vi "Init.vi"(8 "error in (no error)":errorcluster caption="错误输入（无错误）", 10 "Url":string, 11 "HttpClient 输入":refnum<class "HttpClient.lvclass"> caption="DNL_LabVIEW Object in") -> (0 "error out":errorcluster caption="错误输出", 3 "HttpClient 输出":refnum<class "HttpClient.lvclass"> caption="DNL_LabVIEW Object out")   [LabVIEW 2012, in "HttpClient.lvclass"]
uses:
  HttpClient.lvclass
  HttpClient.lvclass/HttpClient.ctl
  Libs/Http/Http.lvclass
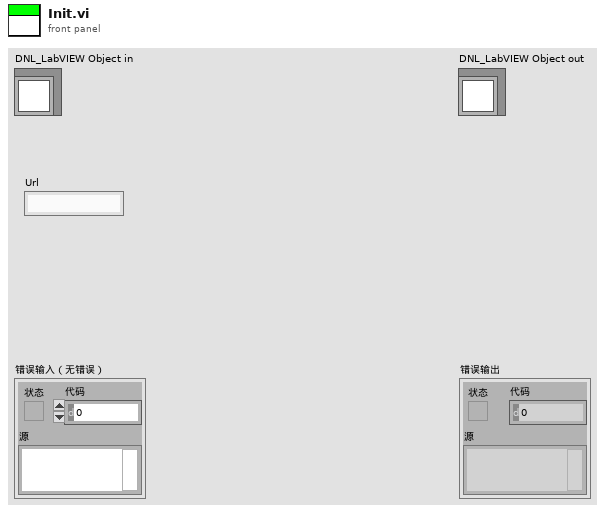
[diagram p1: front panel]
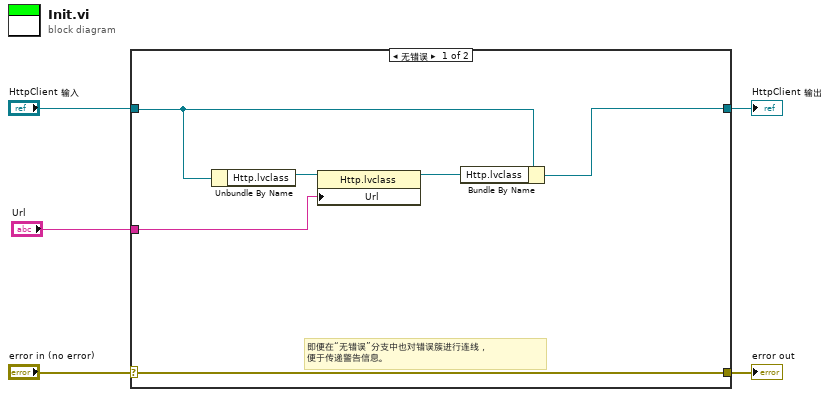
[diagram p0: block diagram]
diagram:
  n1 = case shown="无错误" "error in (no error)" {
    selector: "error in (no error)" -> [w11 w13]
    tunnel: [w11 w13] -> w4
    tunnel: [w6 w12] -> w2
    tunnel: "HttpClient 输入" -> [w10 w12]
    tunnel: "Url" -> [w7 _]
    frame No Error {
      # "即便在“无错误”分支中也对错误簇进行连线，\n便于传递警告信息。"
      n2 = Unbundle By Name(w10) -> ("Http.lvclass"=w9:refnum<class "Http.lvclass">)
      n3 = property class="Http.lvclass"(reference=w9, "Url"=w7) -> (reference out=w8:refnum<class "Http.lvclass">)  [unwired: 1 in, 1 out]
      n4 = Bundle By Name(cluster=w10, "Http.lvclass"=w8) -> (w6:refnum<class "HttpClient.lvclass">)
    }
    frame Error {
    }
  }
  "error out" <- w4
  "HttpClient 输出" <- w2
